vi "Set Delay.vi"(8 "error in (no error)":errorcluster, 9 "Rate (ps/s)":dbl, 10 "Delay (ps)":dbl, 11 "Instrument.Delay in":refnum<class "Instrument.Aerotech.lvclass">) -> (0 "error out":errorcluster, 3 "Instrument.Delay out":refnum<class "Instrument.Aerotech.lvclass">)   [LabVIEW 2016, in "Instrument.Aerotech.lvclass"]
uses:
  Instrument.Aerotech.lvclass
  Instrument.Aerotech.lvclass/Instrument.Aerotech.ctl
  Aerotech-Ensemble-LabVIEW/2010-5.6/Motion/MoveAbsSingle.vi
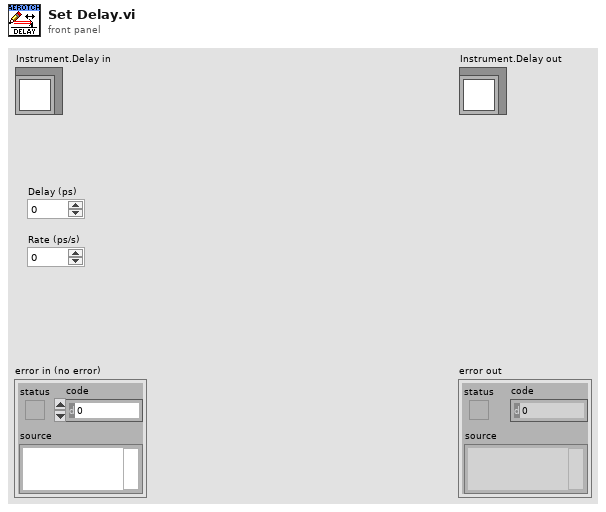
[diagram p1: front panel]
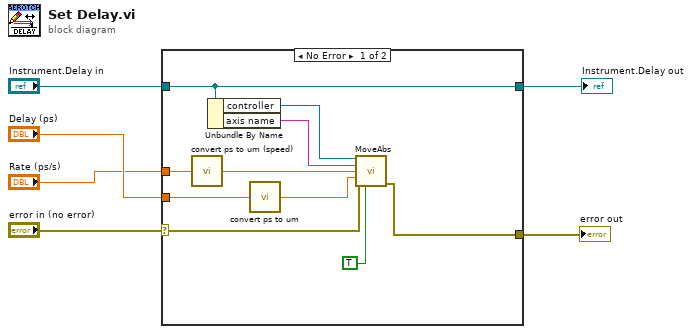
[diagram p0: block diagram]
diagram:
  n1 = case shown="No Error" "error in (no error)" {
    selector: "error in (no error)" -> [w12 w18]
    tunnel: [w16 w18] -> w6
    tunnel: "Delay (ps)" -> [w10 _]
    tunnel: "Rate (ps/s)" -> [w8 _]
    tunnel: "Instrument.Delay in" -> [w11 w17]
    tunnel: [w11 w17] -> w1
    frame No Error {
      n2 = call "convert ps to um (speed).vi"("Delay speed (ps/s)"=w8) -> ("Position speed (um/s)"=w7:dbl)
      n3 = Unbundle By Name(w11) -> ("controller"=w14:refnum<k24>, "axis name"=w13:string)
      n4 = call "convert ps to um.vi"("Delay (ps)"=w10) -> ("Position (um)"=w9:dbl)
      n5 = call-poly "MoveAbs.vi"("controller in"=w14, "axis name"=w13, "speed"=w7, "distance"=w9, "error in (no error)"=w12, "return immediately"=TRUE) -> ("error out"=w16:errorcluster)  [unwired: 8 in, 1 out]
    }
    frame Error {
    }
  }
  "error out" <- w6
  "Instrument.Delay out" <- w1
